vi "SVA_MAIN.vi"() -> ()   [LabVIEW 2021]
panel:
  out "Image Out 3":T1(plugin-control)
  out "Image Out 2":T1(plugin-control)
  in  "Stop":bool
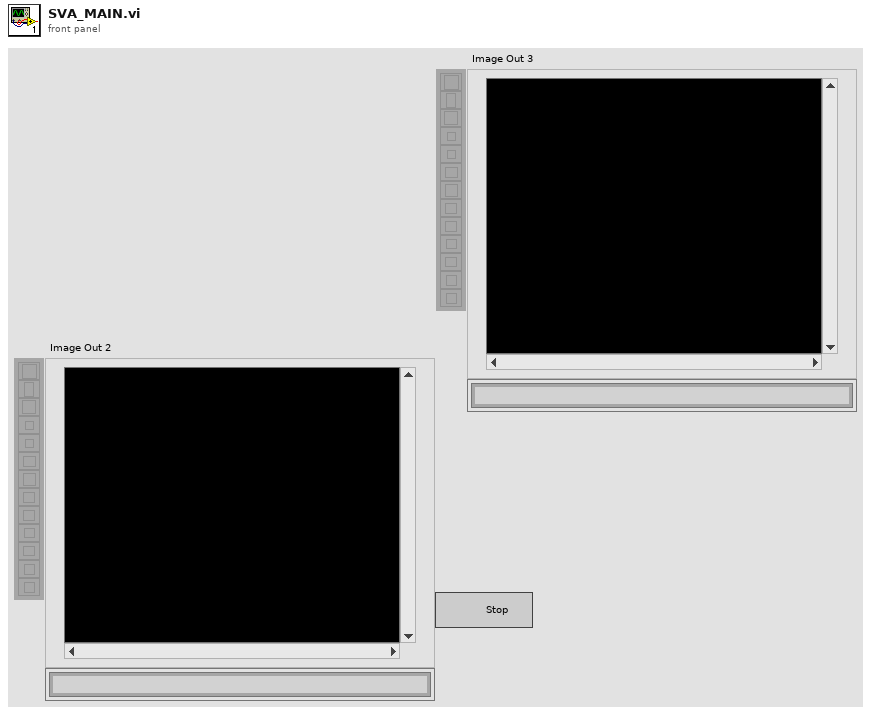
[diagram p1: front panel]
types:
  T1 = typedef "IMAQ Image.ctl" = refnum<image>
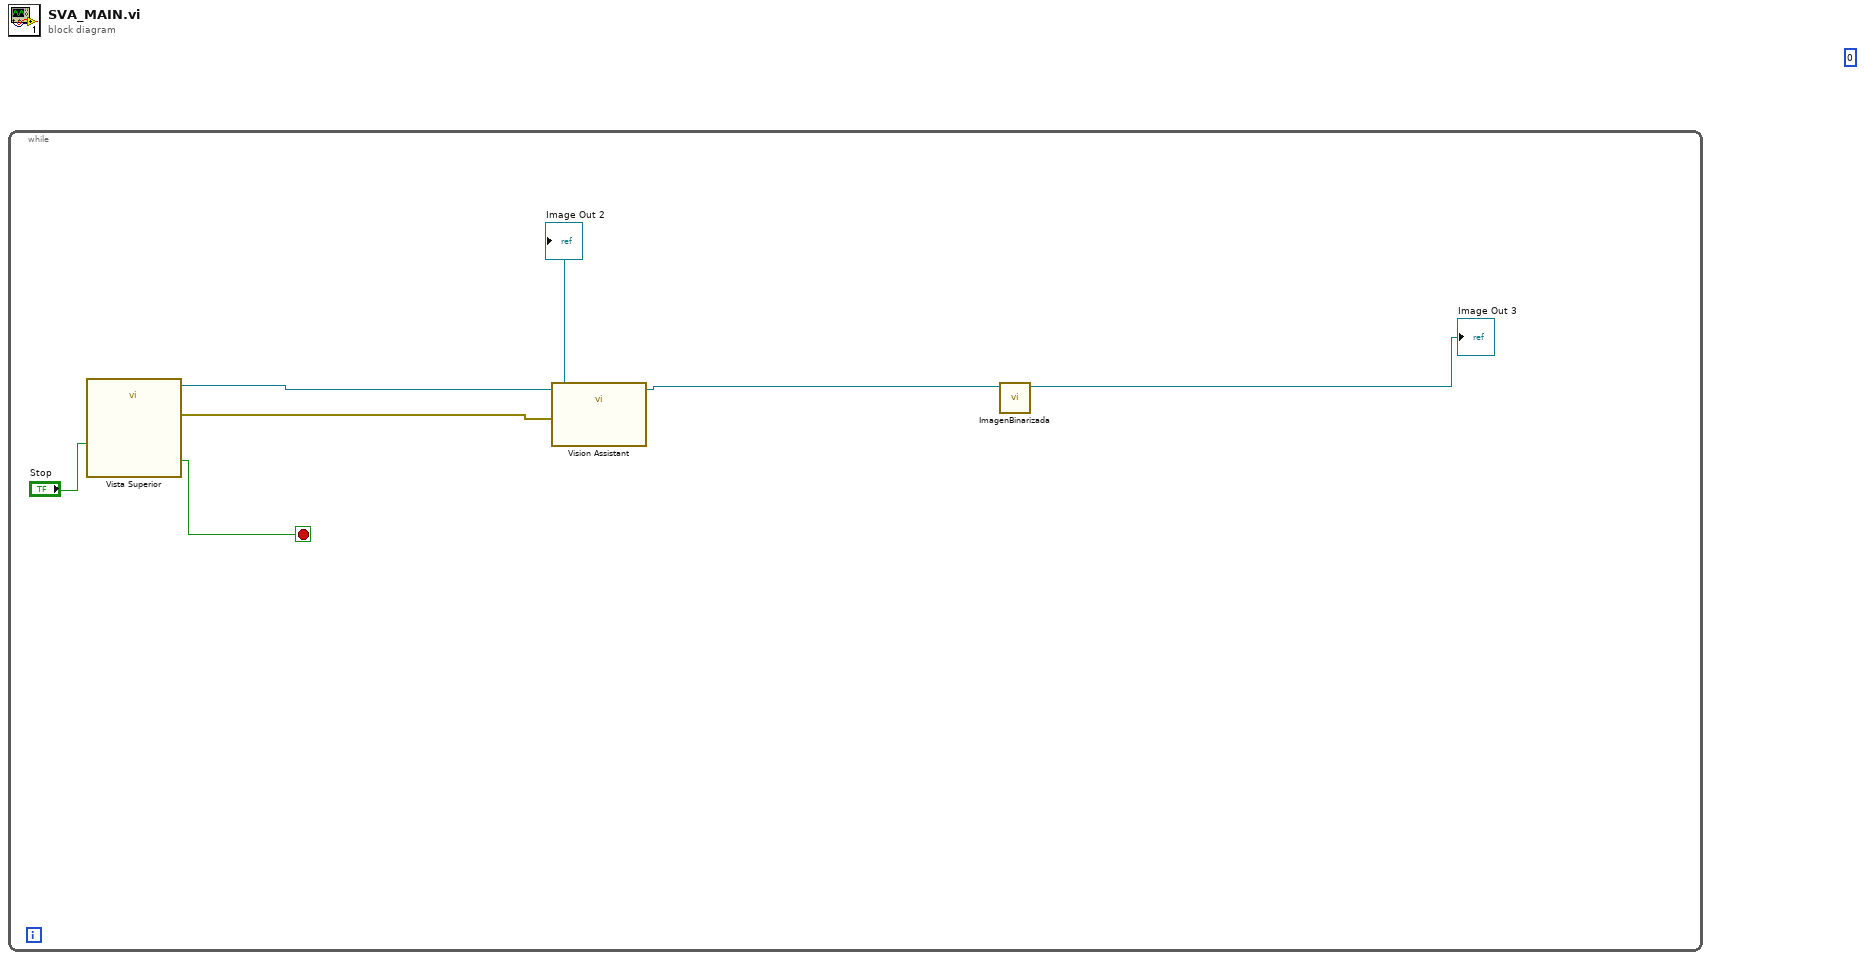
[diagram p0: block diagram]
diagram:
  (unwired) u32 0 ("Bit Depth (0)")
  n1 = while {
    stop <- w5 stop-if-true
    n2 = call "Vista Superior"("Stop (F)"="Stop") -> ("Image Out"=w4:T1, "Stopped"=w5:bool, "error out"=w3:errorcluster)  [unwired: 24 in]
    "Image Out 2" <- w4
    n3 = call "Vision Assistant"("Image In"=w4, "error in"=w3) -> ("Image Out"=w2:T1)  [unwired: 24 in, 1 out]
    n4 = call "ImagenBinarizada.vi"("Refnum in"=w2) -> ("Refnum out"=→"Image Out 3":T1)  [unwired: 10 in]
  }
